vi "dA.vi"() -> ()   [LabVIEW 2012]
uses:
  <vilib>/Analysis/Matrix/Numeric/Conversions/Array To Matrix - RA2.vi
  <vilib>/Analysis/Matrix/Numeric/Conversions/Matrix To Array - RM.vi
  <vilib>/Analysis/Matrix/NI_Matrix.lvlib
panel:
  out "Frequency Num 2":string
  in  "error in 2":errorcluster
  out "error out 2":errorcluster
  out "Frequency Num":string
  out "array 1.0":dbl[][](array[numeric])
  out "array .9":dbl[][](array[numeric])
  out "array .8":dbl[][](array[numeric])
  out "array .7":dbl[][](array[numeric])
  out "array .6":dbl[][](array[numeric])
  out "array .5":dbl[][](array[numeric])
  out "array .4":dbl[][](array[numeric])
  out "array .1":dbl[][](array[numeric])
  out "array .3":dbl[][](array[numeric])
  out "array .2":dbl[][](array[numeric])
  out "divisions":dbl
  in  "Number of Data Sets To Generate":dbl
  out "error out":errorcluster
  in  "F,Vx,Vy,Vr,Phase at Z = 1":path
  in  "F,Vx,Vy,Vr,Phase at Z = .9":path
  in  "F,Vx,Vy,Vr,Phase at Z = .8":path
  in  "F,Vx,Vy,Vr,Phase at Z = .7":path
  in  "F,Vx,Vy,Vr,Phase at Z = .6":path
  in  "F,Vx,Vy,Vr,Phase at Z = .5":path
  in  "F,Vx,Vy,Vr,Phase at Z = .4":path
  in  "F,Vx,Vy,Vr,Phase at Z = .3":path
  in  "F,Vx,Vy,Vr,Phase at Z = .2":path
  in  "F,Vx,Vy,Vr,Phase at Z = .1":path
  out "array 0":dbl[][](array[numeric])
  out "Z-Array":dbl[][](array[numeric])
  in  "error in":errorcluster
  in  "F,Vx,Vy,Vr,Phase at Z = 0":path
  in  "Z Array":path
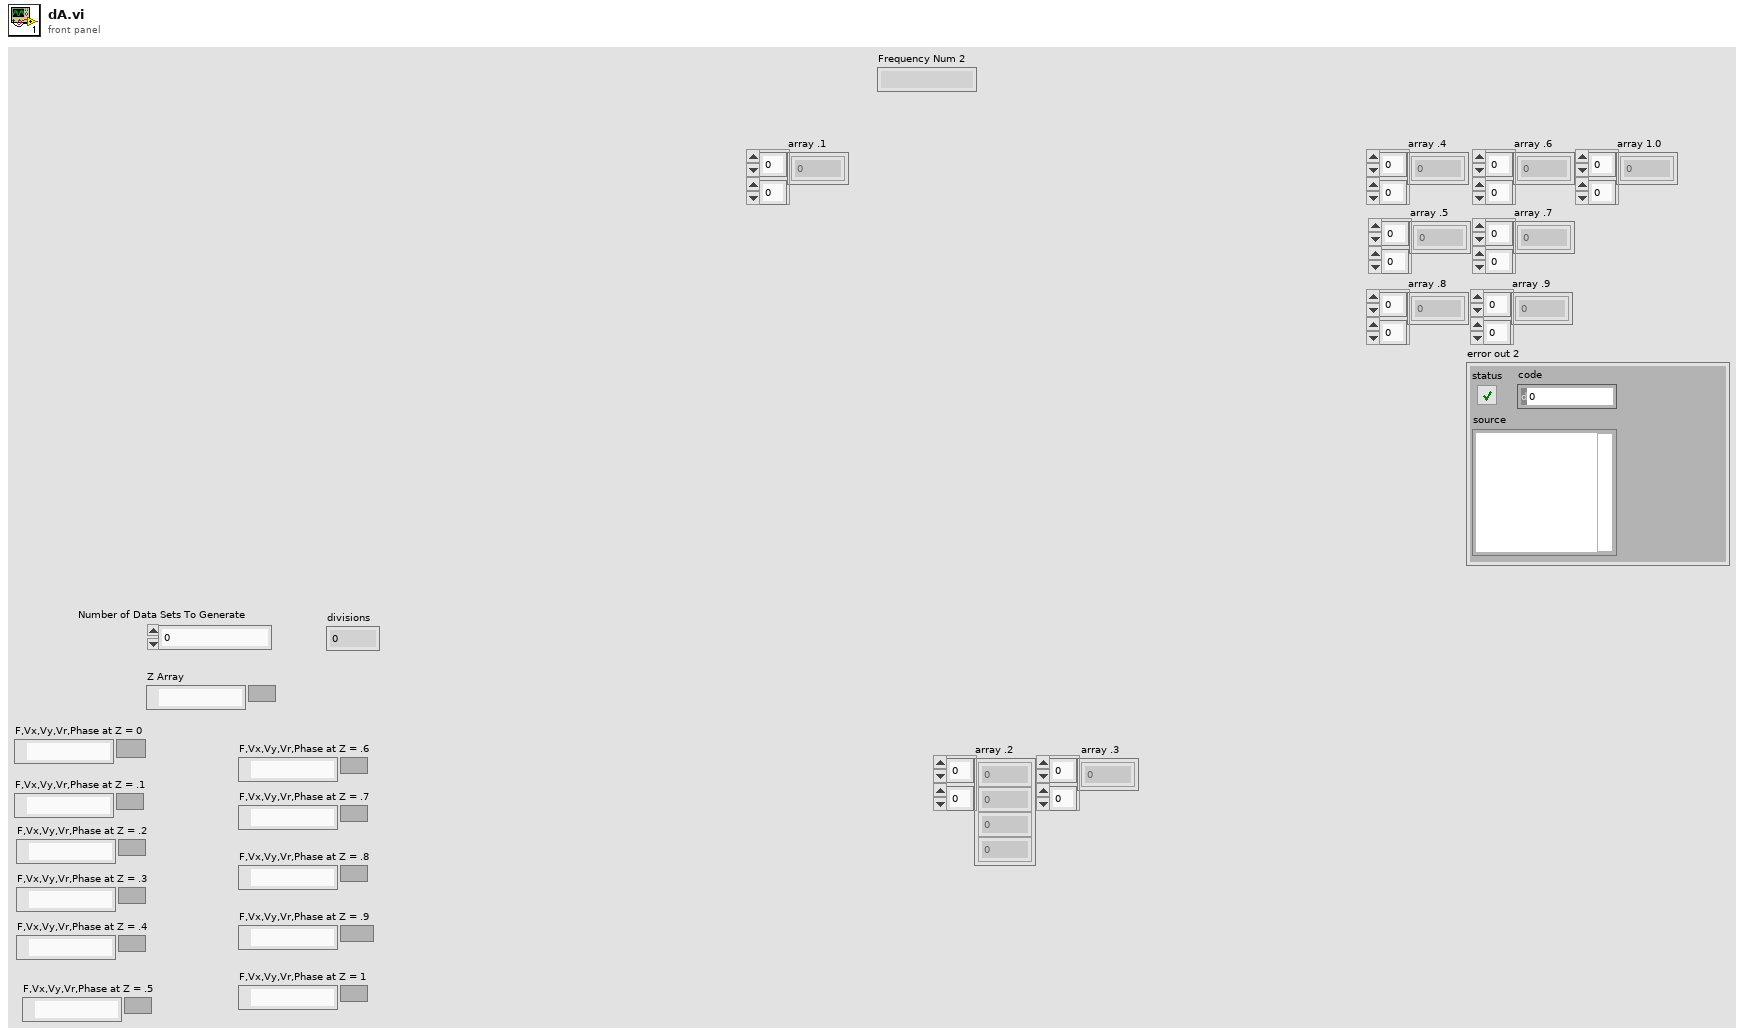
[diagram p1: front panel]
types:
  T1 = typedef "NI_Matrix.lvlib/RealMatrix.ctl" = dbl[][]
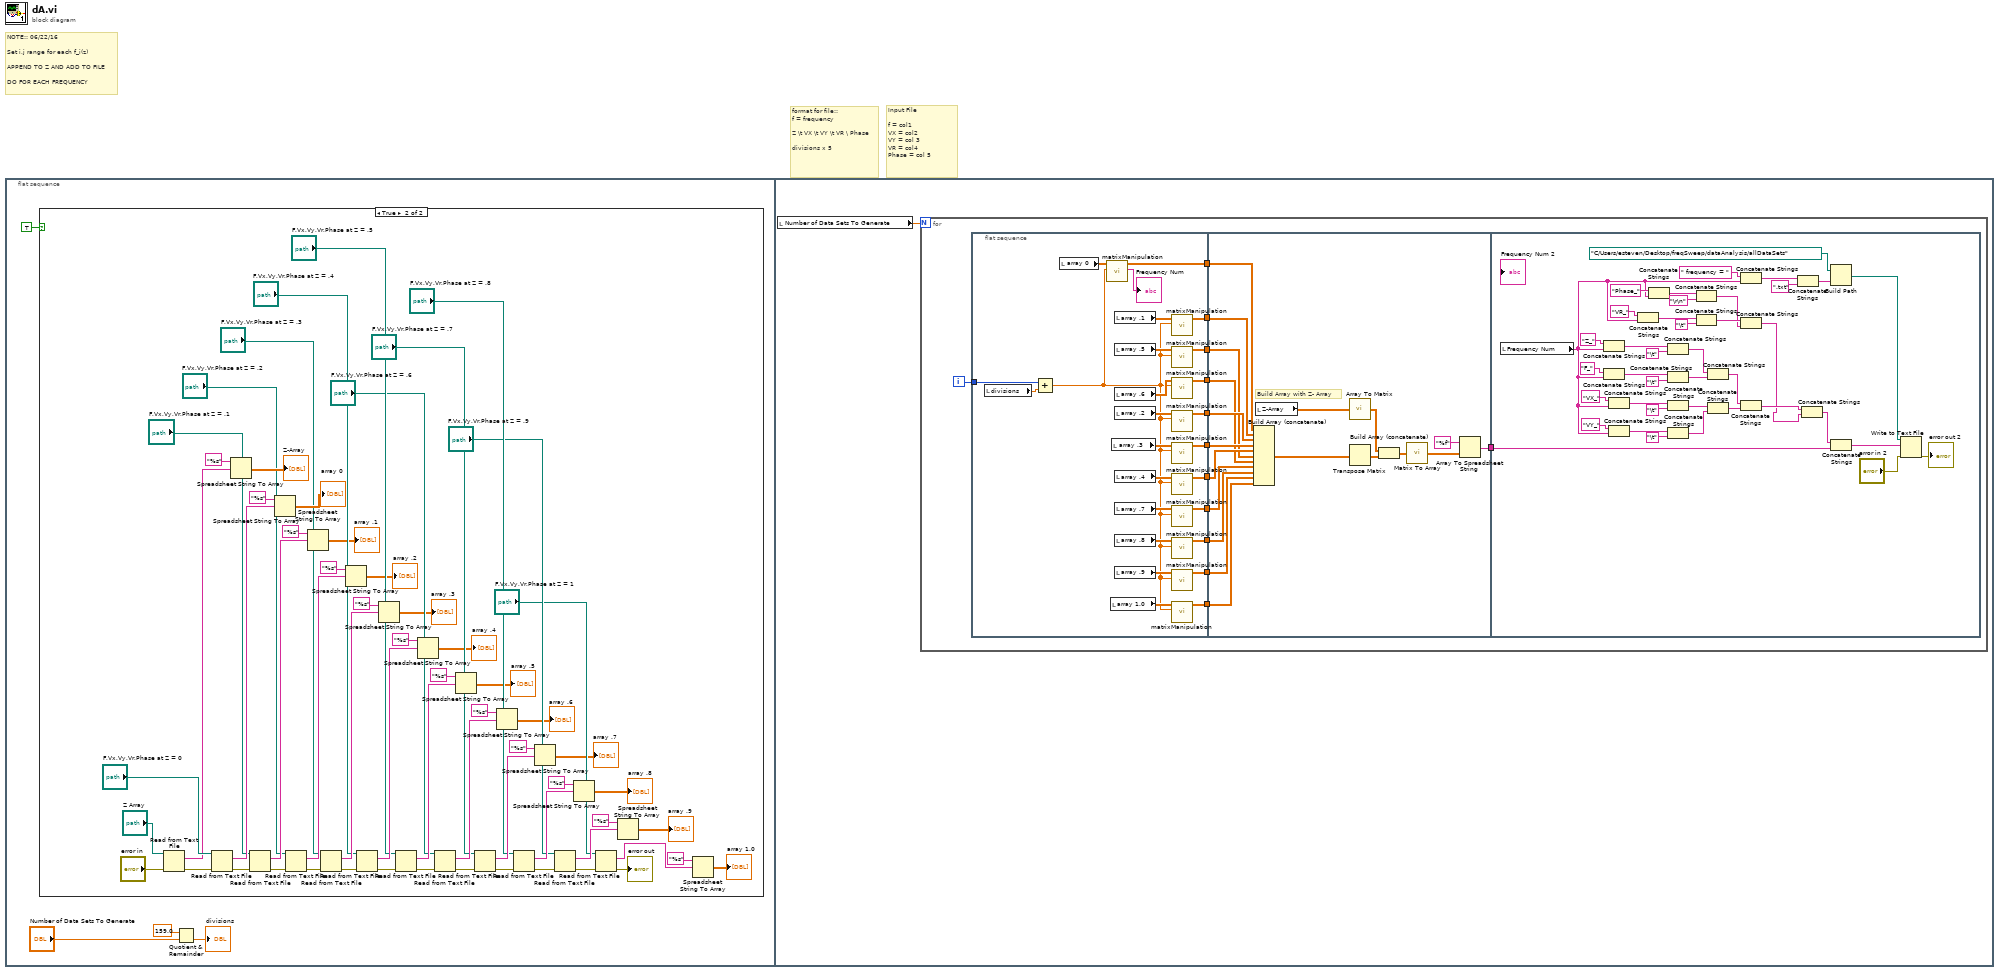
[diagram p0: block diagram]
diagram:
  # "NOTE:: 06/22/16\n\nSet i,j range for each f_i(z) \n\nAPPEND TO Z AND ADD TO FILE \n\nDO FOR EACH FREQUENCY"
  # "Input File \n\nf = col1\nVX = col2\nVY = col 3\nVR = col4\nPhase = col 5"
  # "format for file:: \nf = frequency\n\nZ \\t VX \\t VY \\t VR \\ Phase\n\ndivisions x 5"
  n1 = flat-sequence {
    frame #0 {
      n2 = case shown="True" TRUE {
        frame False {
        }
        frame True {
          n3 = Read from Text File(file (use dialog)="Z Array", error in="error in") -> (text=w62:string, error out=w26:errorcluster)  [unwired: 2 in, 2 out]
          n4 = Read from Text File(file (use dialog)="F,Vx,Vy,Vr,Phase at Z = 0", error in=w26) -> (text=w59:string, error out=w25:errorcluster)  [unwired: 2 in, 2 out]
          n5 = Spreadsheet String To Array(format string="%s", spreadsheet string=w62) -> (array=→"Z-Array":dbl[][])  [unwired: 2 in]
          n6 = Read from Text File(file (use dialog)="F,Vx,Vy,Vr,Phase at Z = .1", error in=w25) -> (text=w54:string, error out=w24:errorcluster)  [unwired: 2 in, 2 out]
          n7 = Spreadsheet String To Array(format string="%s", spreadsheet string=w59) -> (array=→"array 0":dbl[][])  [unwired: 2 in]
          n8 = Read from Text File(file (use dialog)="F,Vx,Vy,Vr,Phase at Z = .2", error in=w24) -> (text=w51:string, error out=w23:errorcluster)  [unwired: 2 in, 2 out]
          n9 = Spreadsheet String To Array(format string="%s", spreadsheet string=w54) -> (array=→"array .1":dbl[][])  [unwired: 2 in]
          n10 = Read from Text File(file (use dialog)="F,Vx,Vy,Vr,Phase at Z = .3", error in=w23) -> (text=w48:string, error out=w22:errorcluster)  [unwired: 2 in, 2 out]
          n11 = Spreadsheet String To Array(format string="%s", spreadsheet string=w51) -> (array=→"array .2":dbl[][])  [unwired: 2 in]
          n12 = Read from Text File(file (use dialog)="F,Vx,Vy,Vr,Phase at Z = .4", error in=w22) -> (text=w45:string, error out=w16:errorcluster)  [unwired: 2 in, 2 out]
          n13 = Spreadsheet String To Array(format string="%s", spreadsheet string=w48) -> (array=→"array .3":dbl[][])  [unwired: 2 in]
          n14 = Read from Text File(file (use dialog)="F,Vx,Vy,Vr,Phase at Z = .5", error in=w16) -> (text=w42:string, error out=w15:errorcluster)  [unwired: 2 in, 2 out]
          n15 = Spreadsheet String To Array(format string="%s", spreadsheet string=w45) -> (array=→"array .4":dbl[][])  [unwired: 2 in]
          n16 = Read from Text File(file (use dialog)="F,Vx,Vy,Vr,Phase at Z = .6", error in=w15) -> (text=w39:string, error out=w21:errorcluster)  [unwired: 2 in, 2 out]
          n17 = Spreadsheet String To Array(format string="%s", spreadsheet string=w42) -> (array=→"array .5":dbl[][])  [unwired: 2 in]
          n18 = Read from Text File(file (use dialog)="F,Vx,Vy,Vr,Phase at Z = .7", error in=w21) -> (text=w36:string, error out=w20:errorcluster)  [unwired: 2 in, 2 out]
          n19 = Spreadsheet String To Array(format string="%s", spreadsheet string=w39) -> (array=→"array .6":dbl[][])  [unwired: 2 in]
          n20 = Read from Text File(file (use dialog)="F,Vx,Vy,Vr,Phase at Z = .8", error in=w20) -> (text=w33:string, error out=w19:errorcluster)  [unwired: 2 in, 2 out]
          n21 = Spreadsheet String To Array(format string="%s", spreadsheet string=w36) -> (array=→"array .7":dbl[][])  [unwired: 2 in]
          n22 = Read from Text File(file (use dialog)="F,Vx,Vy,Vr,Phase at Z = .9", error in=w19) -> (text=w30:string, error out=w18:errorcluster)  [unwired: 2 in, 2 out]
          n23 = Spreadsheet String To Array(format string="%s", spreadsheet string=w33) -> (array=→"array .8":dbl[][])  [unwired: 2 in]
          n24 = Read from Text File(file (use dialog)="F,Vx,Vy,Vr,Phase at Z = 1", error in=w18) -> (text=w27:string, error out=→"error out":errorcluster)  [unwired: 2 in, 2 out]
          n25 = Spreadsheet String To Array(format string="%s", spreadsheet string=w30) -> (array=→"array .9":dbl[][])  [unwired: 2 in]
          n26 = Spreadsheet String To Array(format string="%s", spreadsheet string=w27) -> (array=→"array 1.0":dbl[][])  [unwired: 2 in]
        }
      }
      n27 = Quotient & Remainder(x=159.0, y="Number of Data Sets To Generate") -> (floor(x/y)=→"divisions":dbl)  [unwired: 1 out]
    }
    frame #1 {
      n28 = local read "Number of Data Sets To Generate"() -> (w66:dbl)
      n29 = for {
        N: w66 -> [_]
        i -> [w79]
        n30 = flat-sequence {
          tunnel: w79 -> [w105]
          tunnel: [w91] -> w78
          tunnel: [w90] -> w77
          tunnel: [w89] -> w76
          tunnel: [w88] -> w75
          tunnel: [w87] -> w74
          tunnel: [w86] -> w73
          tunnel: [w85] -> w72
          tunnel: [w84] -> w71
          tunnel: [w83] -> w70
          tunnel: [w82] -> w69
          tunnel: [w81] -> w68
          tunnel: w78 -> [w120]
          tunnel: w77 -> [w119]
          tunnel: w76 -> [w118]
          tunnel: w75 -> [w117]
          tunnel: w74 -> [w116]
          tunnel: w73 -> [w115]
          tunnel: w72 -> [w114]
          tunnel: w71 -> [w113]
          tunnel: w70 -> [w112]
          tunnel: w69 -> [w111]
          tunnel: w68 -> [w110]
          tunnel: [w106] -> w67
          tunnel: w67 -> [w127]
          frame #0 {
            n31 = local read "divisions"() -> (w104:dbl)
            n32 = Add(x=w105, y=w104) -> (x+y=w80:dbl)
            n33 = local read "array 0"() -> (w103:dbl[][])
            n34 = call "matrixManipulation.vi"("J Index"=w80, "Input Array"=w103) -> ("Frequency Num"=→"Frequency Num":string, "Output Array at Frequency Num"=w91:dbl[][])  [unwired: 8 in]
            n35 = local read "array 1.0"() -> (w93:dbl[][])
            n36 = local read "array .3"() -> (w100:dbl[][])
            n37 = local read "array .1"() -> (w102:dbl[][])
            n38 = local read "array .5"() -> (w98:dbl[][])
            n39 = local read "array .6"() -> (w97:dbl[][])
            n40 = local read "array .2"() -> (w101:dbl[][])
            n41 = local read "array .4"() -> (w99:dbl[][])
            n42 = local read "array .7"() -> (w96:dbl[][])
            n43 = local read "array .8"() -> (w95:dbl[][])
            n44 = local read "array .9"() -> (w94:dbl[][])
            n45 = call "matrixManipulation.vi"("J Index"=w80, "Input Array"=w102) -> ("Output Array at Frequency Num"=w90:dbl[][])  [unwired: 8 in, 1 out]
            n46 = call "matrixManipulation.vi"("J Index"=w80, "Input Array"=w98) -> ("Output Array at Frequency Num"=w86:dbl[][])  [unwired: 8 in, 1 out]
            n47 = call "matrixManipulation.vi"("J Index"=w80, "Input Array"=w97) -> ("Output Array at Frequency Num"=w85:dbl[][])  [unwired: 8 in, 1 out]
            n48 = call "matrixManipulation.vi"("J Index"=w80, "Input Array"=w101) -> ("Output Array at Frequency Num"=w89:dbl[][])  [unwired: 8 in, 1 out]
            n49 = call "matrixManipulation.vi"("J Index"=w80, "Input Array"=w100) -> ("Output Array at Frequency Num"=w88:dbl[][])  [unwired: 8 in, 1 out]
            n50 = call "matrixManipulation.vi"("J Index"=w80, "Input Array"=w99) -> ("Output Array at Frequency Num"=w87:dbl[][])  [unwired: 8 in, 1 out]
            n51 = call "matrixManipulation.vi"("J Index"=w80, "Input Array"=w96) -> ("Output Array at Frequency Num"=w84:dbl[][])  [unwired: 8 in, 1 out]
            n52 = call "matrixManipulation.vi"("J Index"=w80, "Input Array"=w95) -> ("Output Array at Frequency Num"=w83:dbl[][])  [unwired: 8 in, 1 out]
            n53 = call "matrixManipulation.vi"("J Index"=w80, "Input Array"=w94) -> ("Output Array at Frequency Num"=w82:dbl[][])  [unwired: 8 in, 1 out]
            n54 = call "matrixManipulation.vi"("J Index"=w80, "Input Array"=w93) -> ("Output Array at Frequency Num"=w81:dbl[][])  [unwired: 8 in, 1 out]
          }
          frame #1 {
            # "Build Array with Z- Array"
            n55 = Build Array (concatenate)(w120, w119, w118, w117, w116, w115, w114, w113, w112, w111, w110) -> (w123:T1)
            n56 = local read "Z-Array"() -> (w124:dbl[][])
            n57 = call-poly <vilib>:"Array To Matrix.vi"("Real 2D Array"=w124) -> ("Real Matrix"=w122:T1)
            n58 = Transpose Matrix(1:w123) -> (0:w121:T1)
            n59 = Build Array (concatenate)(w122, w121) -> (w109:T1)
            n60 = call-poly <vilib>:"Matrix To Array.vi"("Real Matrix"=w109) -> ("Real 2D Array"=w108:dbl[][])
            n61 = Array To Spreadsheet String(array=w108, 3:"%f" ("format string")) -> (spreadsheet string=w106:string)  [unwired: 1 in]
          }
          frame #2 {
            n62 = local read "Frequency Num"() -> (w139:string)
            n63 = Concatenate Strings("F_" ("string"), w139) -> (w151:string)
            n64 = Concatenate Strings("Z_" ("string"), w139) -> (w154:string)
            n65 = Concatenate Strings("VX_" ("string"), w139) -> (w148:string)
            n66 = Concatenate Strings("VY_" ("string"), w139) -> (w142:string)
            n67 = Concatenate Strings("VR_" ("string"), w139) -> (w145:string)
            n68 = Concatenate Strings("Phase_" ("string"), w139) -> (w140:string)
            n69 = Concatenate Strings(w154, "\t") -> (w138:string)
            n70 = Concatenate Strings(w151, "\t") -> (w137:string)
            n71 = Concatenate Strings(w148, "\t") -> (w136:string)
            n72 = Concatenate Strings(w142, "\t") -> (w135:string)
            n73 = Concatenate Strings(w140, "\r\n") -> (w133:string)
            n74 = Concatenate Strings(w145, "\t") -> (w134:string)
            n75 = Concatenate Strings(w138, w137) -> (w131:string)
            n76 = Concatenate Strings(w136, w135) -> (w130:string)
            n77 = Concatenate Strings(" frequency = " ("string"), w139) -> (w162:string)
            n78 = Concatenate Strings(w134, w133) -> (w125:string)
            n79 = Concatenate Strings(w131, w130) -> (w129:string)
            n80 = Concatenate Strings(w162, ".txt" ("string")) -> (w164:string)
            n81 = Concatenate Strings(w129, w125) -> (w128:string)
            n82 = Build Path(base path=path "C:/Users/esteven/Desktop/freqSweep/dataAnalysis/allDataSets", name or relative path=w164) -> (appended path=w157:path)
            n83 = Concatenate Strings(w128, w127) -> (w126:string)
            n84 = Write to Text File(file (use dialog)=w157, text=w126, error in="error in 2") -> (error out=→"error out 2":errorcluster)  [unwired: 1 in, 2 out]
          }
        }
      }
    }
  }
